vi "teleop2.vi"   [LabVIEW 2012, in "Test.lvrbt"]
uses:
  Test.lvrbt
  <vilib>/FTC/FTC Read Controller Packet.vi
  <vilib>/NXT/LegoClasses/BrickReference/BrickReference.lvclass
  <vilib>/NXT/Subs/LVHSConnector.ctl
  <vilib>/NXT/NXTIO Xnodes/NXTIOXNode/NXTIO.xnode
  <vilib>/NXT/NXTIO Xnodes/AddressXNode/NXTIOAddress.xnode
  <vilib>/NXT/Block Support/NXT_OutputPort.ctl
  <vilib>/NXT/Hardware/Plugins/Tetrix DC Motor/TetrixDCMotorAddress.ctl
  <vilib>/NXT/NXTIO Xnodes/NXTIONodeSubVIs/TETRIX IO Move DC Motors.vi
  <vilib>/NXT/NXTIO Xnodes/NXTIONodeSubVIs/NXTMoveMotors.vi
  <vilib>/NXT/NXTIO Xnodes/NXTIONodeSubVIs/NXTStopMotors.vi
  <vilib>/NXT/NXTIO Xnodes/NXTIONodeSubVIs/TETRIX IO Check Battery.vi
  <vilib>/NXT/NXTIO Xnodes/NXTIONodeSubVIs/TETRIX IO Stop DC Motors.vi
  <vilib>/FTC/FTC Interpret Motor Power From Right Y Axis.vi
  <vilib>/FTC/FTC Interpret Motor Power From Left Y Axis.vi
panel:
  # "This VI was generated based on your configuration in the Remote Control Editor. You may modify the code as needed for your robot. To test this program for an FTC match, return to the Remote Control Editor, select the \"Run Program\" tab, and choose \"Teleop\"."
types:
  T1 = typedef "TetrixDCMotorAddress.ctl" = i32
  T2 = cluster{"TetrixDCMotor":T1, "TetrixDCMotor 2":T1}
  T3 = typedef "LVHSConnector.ctl" = refnum<class "BrickReference.lvclass">
  T4 = typedef "FTC ControllerState.ctl" = cluster{"Left X":i8, "Left Y":i8, "Right X":i8, "Right Y":i8, "Button Encoding 9-12":u8, "Button Encoding 1-8":u8, "POV":T5}
  T5 = typedef "FTC POVState.ctl" = i8
  T6 = typedef "FTC ButtonEventType.ctl" = enum16{"Pressed", "Released"}
  T7 = cluster{"Button ID":enum16{"None", "Button 1", "Button 2", "Button 3", "Button 4", "Button 5", "Button 6", "Button 7", "Button 8", "Button 9", "Button 10", "Button 11", "Button 12", "POV Up", "POV Up Right", "POV Right", "POV Down Right", "POV Down", "POV Down Left", "POV Left", "POV Up Left"}, "Event Type":T6}[]
  T8 = enum16{"None", "Button 1", "Button 2", "Button 3", "Button 4", "Button 5", "Button 6", "Button 7", "Button 8", "Button 9", "Button 10", "Button 11", "Button 12", "POV Up", "POV Up Right", "POV Right", "POV Down Right", "POV Down", "POV Down Left", "POV Left", "POV Up Left"}
  T9 = typedef "NXT_OutputPort.ctl" = u8
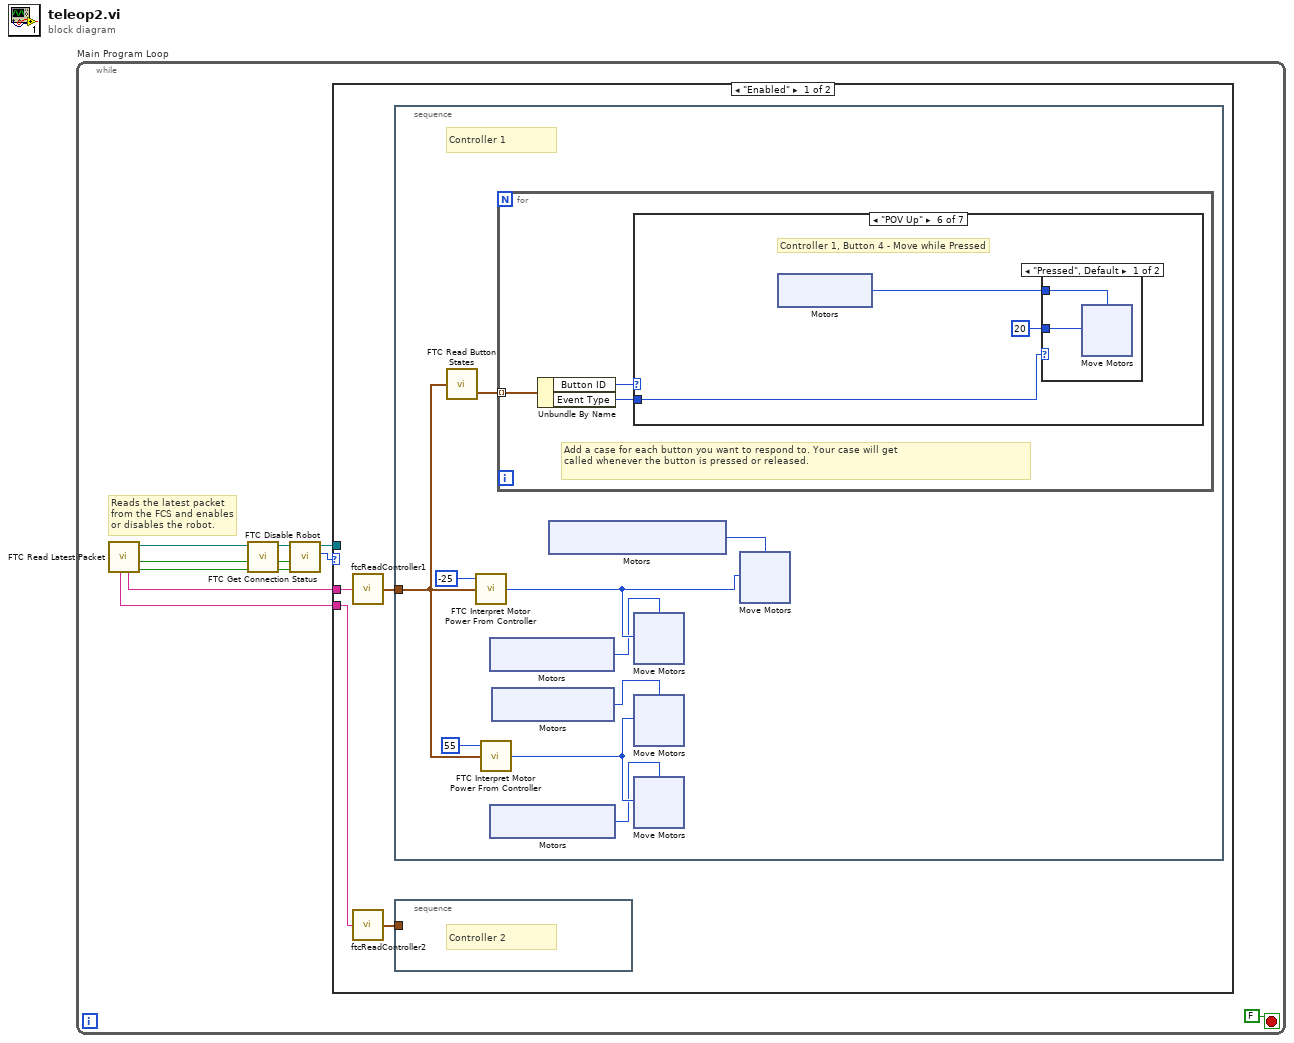
[diagram p0: block diagram]
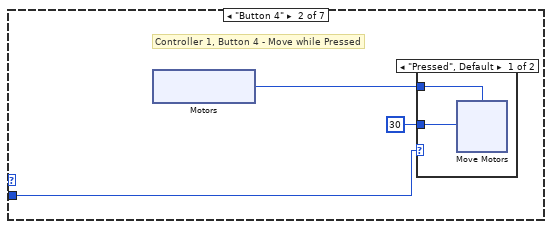
[diagram p3: hidden frame]
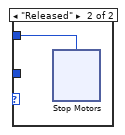
[diagram p4: hidden frame]
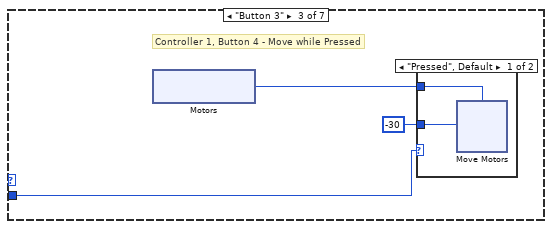
[diagram p5: hidden frame]
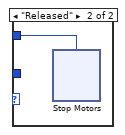
[diagram p6: hidden frame]
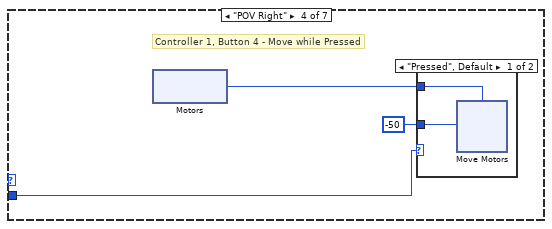
[diagram p7: hidden frame]
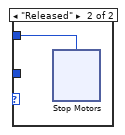
[diagram p8: hidden frame]
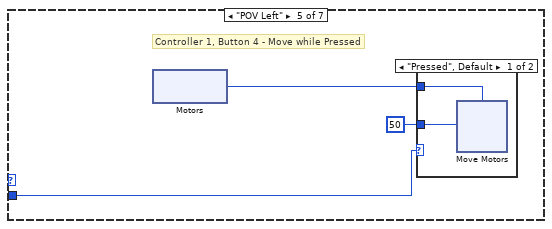
[diagram p9: hidden frame]
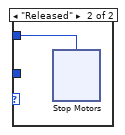
[diagram p10: hidden frame]
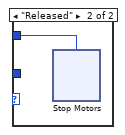
[diagram p11: hidden frame]
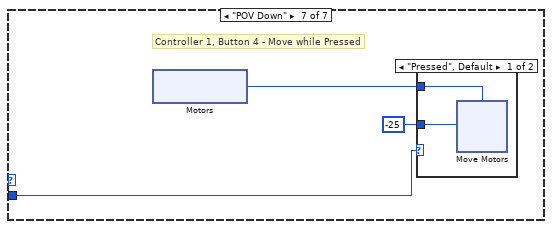
[diagram p12: hidden frame]
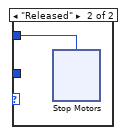
[diagram p13: hidden frame]
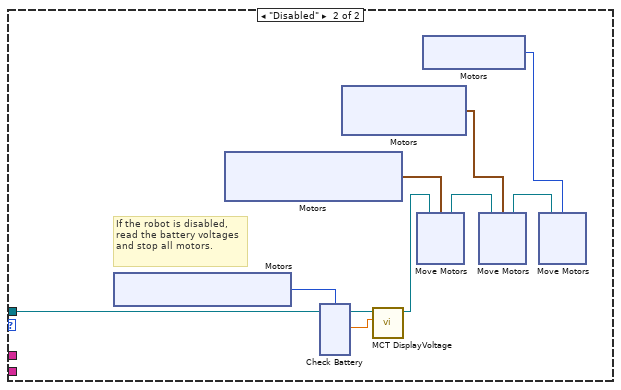
[diagram p14: hidden frame]
diagram:
  n1 = while "Main Program Loop" {
    stop <- FALSE stop-if-true
    # "Reads the latest packet\nfrom the FCS and enables\nor disables the robot."
    n2 = call <vilib>:"FTC Read Latest Packet.vi"() -> ("Packet Received?"=w8:bool, "Stopped?"=w5:bool, "NXT/EV3"=w7:T3, "Controller 1"=w10:string, "Controller 2"=w9:string)  [unwired: 6 in, 1 out]
    n3 = call <vilib>:"FTC Get Connection Status.vi"("Packet Received?"=w8, "Stopped?"=w5, "NXT/EV3"=w7) -> ("Online?"=w2:bool, "Stopped?"=w3:bool, "NXT/EV3"=w4:T3)  [unwired: 5 in]
    n4 = call <vilib>:"FTC Disable Robot.vi"("Online?"=w2, "Stopped?"=w3, "NXT/EV3"=w4) -> ("Enabled?"=w6:enum16{"Disabled", "Enabled"}, "NXT/EV3"=w1:T3)  [unwired: 3 in]
    n5 = case "disableCase" shown="\"Enabled\"" w6 {
      tunnel: w10 -> [w15 _]
      tunnel: w9 -> [w14 _]
      tunnel: w1 -> [_ w184]
      frame "Enabled" {
        n6 = call "ftcReadController1"("Packet"=w15) -> ("Controller State"=w13:T4)  [unwired: 4 in]
        n7 = call "ftcReadController2"("Packet"=w14) -> ("Controller State"=w12:T4)  [unwired: 4 in]
        n8 = stacked-sequence "controller1Actions" {
          tunnel: w13 -> [w24]
          frame #0 {
            # "Controller 1"
            n9 = call <vilib>:"FTC Read Button States.vi"("Controller State"=w24) -> ("Button Events"=w25:T7)  [unwired: 2 in, 1 out]
            n10 = call-poly <vilib>:"FTC Interpret Motor Power From Controller.vi"("Controller State"=w24, "Power Level (50)"=i8 -25) -> ("Power"=w20:i8)  [unwired: 1 in]
            n11 = call-poly <vilib>:"FTC Interpret Motor Power From Controller.vi"("Controller State"=w24, "Power Level (50)"=i8 55) -> ("Power"=w19:i8)  [unwired: 1 in]
            n12 = xnode "Motors"() -> ("Motor"=w18:T1)
            n13 = xnode "Motors"() -> ("Motor"=w17:T1)
            n14 = xnode ("Motors")() -> ("Motor"=w16:T1)
            n15 = for "buttonAction" {
              tunnel: w25 -> [w58] mode=indexing
              # "Add a case for each button you want to respond to. Your case will get \ncalled whenever the button is pressed or released."
              n16 = Unbundle By Name(w58) -> ("Button ID"=w60:T8, "Event Type"=w59:T6)
              n17 = case "EventCase1" shown="\"POV Up\"" w60 {
                tunnel: w59 -> [_ w63 w82 w101 w120 w139 w158]
                frame Default {
                  # "No Action"
                }
                frame "Button 4" {
                  # "Controller 1, Button 4 - Move while Pressed"
                  n18 = xnode "Motors"() -> ("Motor"=w61:T9)
                  n19 = case shown="\"Pressed\", Default" w63 {
                    tunnel: 30 ("Power (75)") -> [w66 _]
                    tunnel: w61 -> [w65 w74]
                    frame "Pressed", Default {
                      n20 = xnode "Move Motors"("Power/Speed 1"=w66, "Motors"=w65) -> ()  [unwired: 1 in, 1 out]
                    }
                    frame "Released" {
                      n21 = xnode "Stop Motors"("Motors"=w74) -> ()  [unwired: 1 in, 1 out]
                    }
                  }
                }
                frame "Button 3" {
                  # "Controller 1, Button 4 - Move while Pressed"
                  n22 = xnode "Motors"() -> ("Motor"=w80:T9)
                  n23 = case shown="\"Pressed\", Default" w82 {
                    tunnel: -30 ("Power (75)") -> [w85 _]
                    tunnel: w80 -> [w84 w93]
                    frame "Pressed", Default {
                      n24 = xnode "Move Motors"("Power/Speed 1"=w85, "Motors"=w84) -> ()  [unwired: 1 in, 1 out]
                    }
                    frame "Released" {
                      n25 = xnode "Stop Motors"("Motors"=w93) -> ()  [unwired: 1 in, 1 out]
                    }
                  }
                }
                frame "POV Right" {
                  # "Controller 1, Button 4 - Move while Pressed"
                  n26 = xnode "Motors"() -> ("Motor"=w99:T1)
                  n27 = case shown="\"Pressed\", Default" w101 {
                    tunnel: -50 ("Power (75)") -> [w104 _]
                    tunnel: w99 -> [w103 w112]
                    frame "Pressed", Default {
                      n28 = xnode "Move Motors"("Power/Speed 1"=w104, "Motors"=w103) -> ()  [unwired: 1 in, 1 out]
                    }
                    frame "Released" {
                      n29 = xnode "Stop Motors"("Motors"=w112) -> ()  [unwired: 1 in, 1 out]
                    }
                  }
                }
                frame "POV Left" {
                  # "Controller 1, Button 4 - Move while Pressed"
                  n30 = xnode "Motors"() -> ("Motor"=w118:T1)
                  n31 = case shown="\"Pressed\", Default" w120 {
                    tunnel: 50 ("Power (75)") -> [w123 _]
                    tunnel: w118 -> [w122 w131]
                    frame "Pressed", Default {
                      n32 = xnode "Move Motors"("Power/Speed 1"=w123, "Motors"=w122) -> ()  [unwired: 1 in, 1 out]
                    }
                    frame "Released" {
                      n33 = xnode "Stop Motors"("Motors"=w131) -> ()  [unwired: 1 in, 1 out]
                    }
                  }
                }
                frame "POV Up" {
                  # "Controller 1, Button 4 - Move while Pressed"
                  n34 = xnode "Motors"() -> ("Motor"=w137:T1)
                  n35 = case shown="\"Pressed\", Default" w139 {
                    tunnel: 20 ("Power (75)") -> [w142 _]
                    tunnel: w137 -> [w141 w150]
                    frame "Pressed", Default {
                      n36 = xnode "Move Motors"("Power/Speed 1"=w142, "Motors"=w141) -> ()  [unwired: 1 in, 1 out]
                    }
                    frame "Released" {
                      n37 = xnode "Stop Motors"("Motors"=w150) -> ()  [unwired: 1 in, 1 out]
                    }
                  }
                }
                frame "POV Down" {
                  # "Controller 1, Button 4 - Move while Pressed"
                  n38 = xnode "Motors"() -> ("Motor"=w156:T1)
                  n39 = case shown="\"Pressed\", Default" w158 {
                    tunnel: -25 ("Power (75)") -> [w161 _]
                    tunnel: w156 -> [w160 w169]
                    frame "Pressed", Default {
                      n40 = xnode "Move Motors"("Power/Speed 1"=w161, "Motors"=w160) -> ()  [unwired: 1 in, 1 out]
                    }
                    frame "Released" {
                      n41 = xnode "Stop Motors"("Motors"=w169) -> ()  [unwired: 1 in, 1 out]
                    }
                  }
                }
              }
            }
            n42 = xnode "Motors"() -> ("Motor"=w21:T1)
            n43 = xnode "Move Motors"("Power/Speed 1"=w20, "Motors"=w18) -> ()  [unwired: 1 in, 1 out]
            n44 = xnode ("Move Motors")("Power/Speed 1"=w19, "Motors"=w16) -> ()  [unwired: 1 in, 1 out]
            n45 = xnode "Move Motors"("Power/Speed 1"=w19, "Motors"=w17) -> ()  [unwired: 1 in, 1 out]
            n46 = xnode "Move Motors"("Power/Speed 1"=w20, "Motors"=w21) -> ()  [unwired: 1 in, 1 out]
          }
        }
        n47 = stacked-sequence "controller2Actions" {
          tunnel: w12 -> [_]
          frame #0 {
            # "Controller 2"
          }
        }
      }
      frame "Disabled" {
        # "If the robot is disabled, read the battery voltages and stop all motors."
        n48 = xnode ("Motors")() -> ("Motor"=w183:T1)
        n49 = xnode "Motors"() -> ("Motor"=w180:cluster{"TetrixDCMotor":T1, "TetrixDCMotor":T1})
        n50 = xnode ("Check Battery")("Motors"=w183, "NXT/EV3"=w184) -> ("Voltage 1"=w182:sgl, "NXT/EV3"=w181:T3)
        n51 = xnode "Motors"() -> ("Motor"=w178:cluster{"TetrixDCMotor":T1, "TetrixDCMotor":T1})
        n52 = call <vilib>:"MCT DisplayVoltage.vi"("Motor Voltage"=w182, "NXT/EV3"=w181) -> ("NXT/EV3"=w179:T3)  [unwired: 9 in]
        n53 = xnode "Move Motors"("Motors"=w180, "NXT/EV3"=w179) -> ("NXT/EV3"=w177:T3)
        n54 = xnode "Motors"() -> ("Motor"=w176:T9)
        n55 = xnode "Move Motors"("Motors"=w178, "NXT/EV3"=w177) -> ("NXT/EV3"=w175:T3)
        n56 = xnode "Move Motors"("Motors"=w176, "NXT/EV3"=w175) -> ()  [unwired: 1 out]
      }
    }
  }
